vi "Configure Acquisition.vi"(8 "error in":errorcluster, 11 "SDS1022 Base CFG in":refnum<class "SDS1022 Base CFG.lvclass">) -> (0 "error out":errorcluster, 3 "SDS1022 Base CFG out":refnum<class "SDS1022 Base CFG.lvclass">)   [LabVIEW 2023, in "OWON SDS1022.lvlib" / "SDS1022 Base CFG.lvclass"]
uses:
  SDS1022 Base CFG.lvclass
  SDS1022 Base CFG.lvclass/SDS1022 Base CFG.ctl
  <instrlib>/OWON SDS1022/OWON SDS1022 Driver.lvlib
  HAL/Configuration Base/Configuration Base.lvclass
  <vilib>/JDP Science/JSONtext/JSONtext.lvlib
  HAL/Scope VISA/Configuration/Scope VISA CFG.lvclass
  D:/git/HAL/Scope VISA/Configuration/Scope VISA CFG.lvclass
  D:/git/HAL/Configuration Base/Configuration Base.lvclass
  D:/git/HAL/Interfaces/IConfigure/IConfigure.lvclass
  D:/git/HAL/Interfaces/IConfigure Scope/IConfigure Scope.lvclass
  D:/git/OWON-SDS1022-LabVIEW/OWON SDS1022/Configurations/SDS1000 Base CFG/SDS1022 Base CFG.lvclass
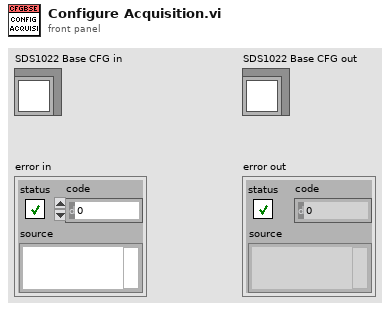
[diagram p1: front panel]
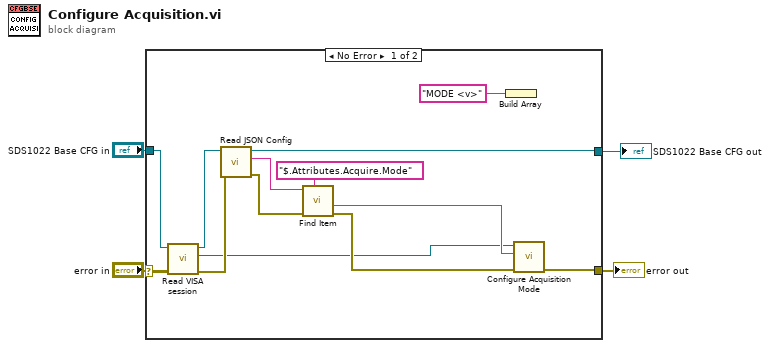
[diagram p0: block diagram]
diagram:
  n1 = case shown="No Error" "error in" {
    selector: "error in" -> [w16 w19]
    tunnel: [w11 w19] -> w4
    tunnel: [w15 w18] -> w3
    tunnel: "SDS1022 Base CFG in" -> [w7 w18]
    frame No Error {
      n2 = call "Read VISA session.vi"("error in (no error)"=w16, "Scope VISA CFG in"=w7) -> ("error out"=w8:errorcluster, "VISA session"=w5:refnum<visa-resource-name>, "Scope VISA CFG out"=w6:refnum<class "SDS1022 Base CFG.lvclass">)  [unwired: 7 in]
      n3 = call "Read JSON Config.vi"("error in"=w8, "object in"=w6) -> ("error out"=w14:errorcluster, "<JSON>Config"=w12:string, "object out"=w15:refnum<class "SDS1022 Base CFG.lvclass">)  [unwired: 7 in]
      n4 = call <vilib>:"Find Item.vi"("$Path or Item Name"="$.Attributes.Acquire.Mode" ("JSON  Path"), "error in (no error)"=w14, "JSON"=w12) -> ("error out"=w10:errorcluster, "<JSON>"=w9:string)  [unwired: 5 in, 2 out]
      n5 = Build Array("MODE <v>") -> ()  [unwired: 1 out]
      n6 = call <instrlib>:"Configure Acquisition Mode.vi"("error in"=w10, "Acquisition Mode (Sample)"=w9, "VISA resource name"=w5) -> ("error out"=w11:errorcluster)  [unwired: 7 in, 1 out]
    }
    frame Error {
    }
  }
  "error out" <- w4
  "SDS1022 Base CFG out" <- w3
